vi "Add Bitfile Dialog.vi"(8 "error in (no error)":errorcluster, 11 "Item Ref in":T1 format="%.0x") -> (0 "error out":errorcluster, 1 "RIO Device Address out":string, 2 "Bitfile Path out":path, 3 "Item Ref out":T1 format="%.0x", 5 "OK?":bool)   [LabVIEW 2015, in "Engine Simulation Toolkit System Explorer.lvlib"]
uses:
  Engine Simulation Toolkit System Explorer.lvlib
  <vilib>/NI Veristand/Custom Device API/Custom Device Item Ref.ctl
  Shared/Properties.vi
  <vilib>/NI Veristand/Custom Device API/Get Item Property (String Array).vi
  <vilib>/NI VeriStand/Custom Device API/Custom Device API.lvlib
  Shared/Engine Simulation Toolkit Shared.lvlib
panel:
  in  "Warning text":string
  in  "Cancel":bool
  in  "OK":bool
  in  "RIO Device Address":string
  in  "Bitfile Path":path
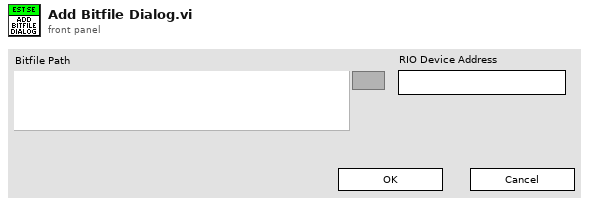
[diagram p1: front panel]
types:
  T1 = typedef "Custom Device API.lvlib/Custom Device Item Ref.ctl" = u64
  T2 = enum8{"Enabled", "Disabled", "Disabled and Grayed Out"}
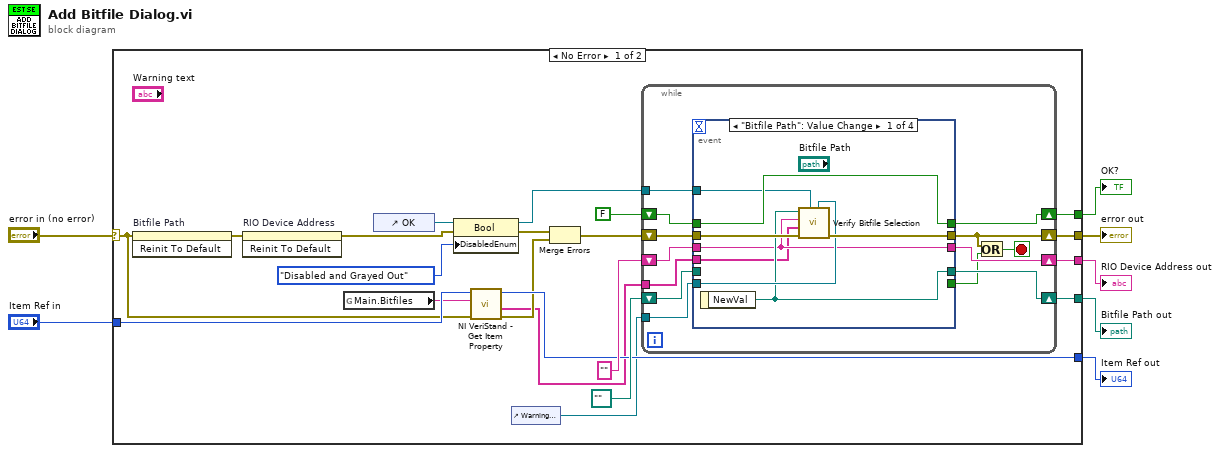
[diagram p0: block diagram]
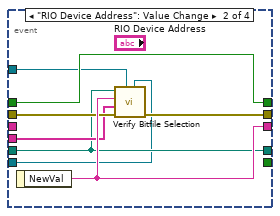
[diagram p2: hidden frame]
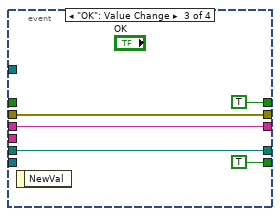
[diagram p3: hidden frame]
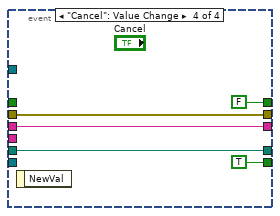
[diagram p4: hidden frame]
diagram:
  n1 = case shown="No Error" "error in (no error)" {
    selector: "error in (no error)" -> [w14 w69]
    tunnel: [w17 w69] -> w7
    tunnel: [w21 _] -> w5
    tunnel: [w20 _] -> w4
    tunnel: [w19 _] -> w3
    tunnel: "Item Ref in" -> [w16 w68]
    tunnel: [w15 w68] -> w1
    frame No Error {
      n2 = invoke on="Bitfile Path" class="Path" method="Reinit To Default"(error in=w14) -> (error out=w28:errorcluster)  [unwired: 2 in, 2 out]
      n3 = invoke on="RIO Device Address" class="Str" method="Reinit To Default"(error in=w28) -> (error out=w18:errorcluster)  [unwired: 2 in, 2 out]
      n4 = global read "Properties.vi" "Main.Bitfiles"() -> (w10:string)
      n5 = control-ref of="OK"() -> (w26:refnum<vi>)
      n6 = property class="Bool"(reference=w26, error in=w18, "DisabledEnum"=T2."Disabled and Grayed Out" ("Disabled")) -> (reference out=w27:refnum<vi>, error out=w13:errorcluster)
      n7 = call-poly <vilib>:"NI VeriStand - Get Item Property.vi"("error in (no error)"=w14, "Property Name"=w10, "Item Ref in"=w16) -> ("error out"=w12:errorcluster, "Value"=w9:string[], "Item Ref out"=w15:T1)  [unwired: 5 in, 1 out]
      n8 = control-ref of="Warning text"() -> (w8:refnum<vi>)
      n9 = Merge Errors(w13, w12) -> (w11:errorcluster)
      n10 = while {
        shift-right: [w39] -> w21
        shift-left: path "" ("NewVal") -> [w37]
        shift-right: [w40] -> w20
        shift-left: "" ("NewVal") -> [w38]
        shift-right: [w41] -> w19
        shift-left: FALSE -> [w36]
        tunnel: w27 -> [w35]
        shift-right: [w31] -> w17
        shift-left: w11 -> [w32]
        tunnel: w9 -> [w29]
        tunnel: w8 -> [w30]
        stop <- w34 stop-if-true
        n11 = event shown="[0] \"Bitfile Path\": Value Change" {
          selector: _ -> [_ _ _ _]
          dyn-events: _ -> [_ _ _ _]
          timeout: _ -> [_ _ _ _]
          tunnel: [_ _ TRUE TRUE] -> w33
          tunnel: [w43 w56 w59 w65] -> w40
          tunnel: [w44 w52 w60 w64] -> w39
          tunnel: [w49 w57 TRUE FALSE] -> w41
          tunnel: w38 -> [w43 _ w59 w65]
          tunnel: w37 -> [_ w52 w60 w64]
          tunnel: w36 -> [w49 w57 _ _]
          tunnel: w35 -> [w46 w51 _ _]
          tunnel: w32 -> [w48 w55 w58 w63]
          tunnel: [w47 w54 w58 w63] -> w31
          tunnel: w30 -> [w45 w50 _ _]
          tunnel: w29 -> [w42 w53 _ _]
          event "Bitfile Path": Value Change {
            n12 = event-data() -> ("NewVal"=w44:path)  [unwired: 1 in]
            n13 = call "Verify Bitfile Selection.vi"("Warning text reference"=w45, "ok button reference in"=w46, "error in (no error)"=w48, "Existing RIO Device Addresses"=w42, "RIO Device Address"=w43, "file path"=w44) -> ("error out"=w47:errorcluster)  [unwired: 5 in]
          }
          event "RIO Device Address": Value Change {
            n14 = event-data() -> ("NewVal"=w56:string)  [unwired: 1 in]
            n15 = call "Verify Bitfile Selection.vi"("Warning text reference"=w50, "ok button reference in"=w51, "error in (no error)"=w55, "Existing RIO Device Addresses"=w53, "RIO Device Address"=w56, "file path"=w52) -> ("error out"=w54:errorcluster)  [unwired: 5 in]
          }
          event "OK": Value Change {
            n16 = event-data() -> ()  [unwired: 1 in, 1 out]
          }
          event "Cancel": Value Change {
            n17 = event-data() -> ()  [unwired: 1 in, 1 out]
          }
        }
        n18 = Or(x=w31, y=w33) -> (x .or. y?=w34:bool)
      }
    }
    frame Error {
    }
  }
  "error out" <- w7
  "OK?" <- w3
  "RIO Device Address out" <- w4
  "Bitfile Path out" <- w5
  "Item Ref out" <- w1
